vi "API BARINIT.vi"() -> (2 "DevInit Return Value":bool)   [LabVIEW 2011, in "API READBC.lvlib"]
uses:
  API READBC.lvlib
  BarCodeAPI.dll
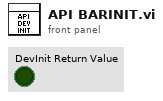
[diagram p1: front panel]
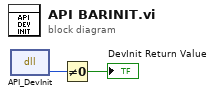
[diagram p0: block diagram]
diagram:
  n1 = dll-call lib="PTH1oabs CUsers\nAdministratorDesktop可重构机电平台项目DemoLabView基础APIBarCodeAPI.dll" fn="API_DevInit"() -> ("返回类型"=w2:i32)  [unwired: 3 in, 2 out]
  n2 = Not Equal To 0?(x=w2) -> (x != 0?=→"DevInit Return Value":bool)
